vi "Dashboard Main.vi"() -> ()   [LabVIEW 2012]
uses:
  <vilib>/Rock Robotics/WPI/Camera/WPI_CameraImageSize.ctl
panel:
  out "Camera Image 3":T1(plugin-control)
  out "Camera Image":T1(plugin-control)
  # "Gatherer Camera"
  # "Shooter Camera"
  # "Team 195 - The CyberKnights"
  # "Screaming Knight Dashboard - 2012"
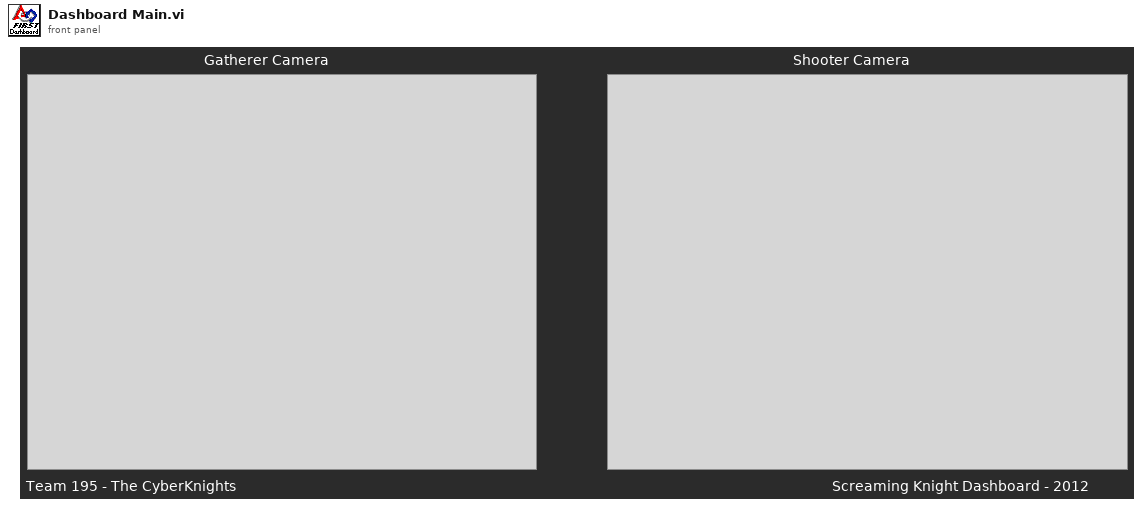
[diagram p1: front panel]
types:
  T1 = typedef "IMAQ Image.ctl" = refnum<image>
  T2 = typedef "Image Type" = u32
  T3 = typedef "WPI_CameraImageSize.ctl" = enum16{"640x480", "320x240", "160x120"}
  T4 = cluster{"fps":i32, "compression":i32, "Image Size":T3}
  T5 = cluster{"Desired Font (Application)":enum16{"User-specified Font", "Application Font", "System Font", "Dialog Font"}, "[User-specified Font]":cluster{"Font Name":string, "Size":i16, "Strikeout?":bool, "Italic?":bool, "Underline?":bool, "Outline?":bool, "Shadow?":bool, "Bold?":bool, "Rotation Angle":dbl}, "Horizontal Alignment":i16, "Vertical Alignment":i16}
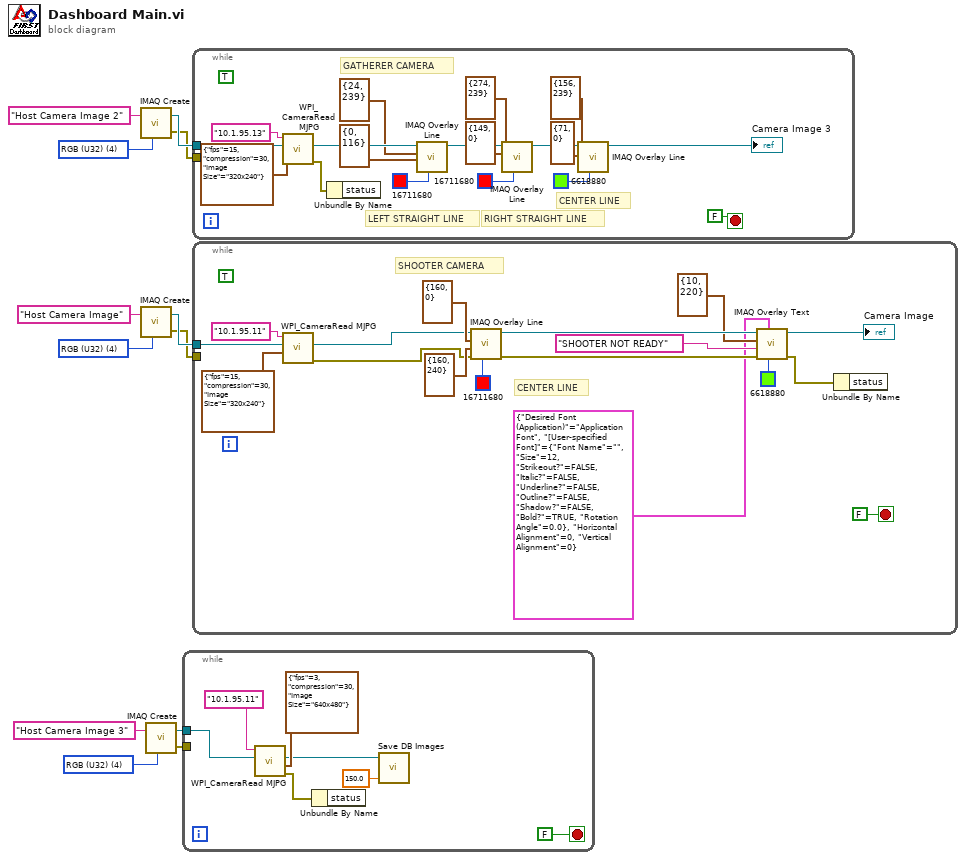
[diagram p0: block diagram]
diagram:
  w4 = T2 4 items=["Grayscale (U8)", "Grayscale (I16)", "Grayscale (SGL)", "Complex (CSG)", "RGB (U32)", "HSL (U32)", "RGB (U64)"] ("Image Type")
  w8 = T2 4 items=["Grayscale (U8)", "Grayscale (I16)", "Grayscale (SGL)", "Complex (CSG)", "RGB (U32)", "HSL (U32)", "RGB (U64)"] ("Image Type")
  w12 = T2 4 items=["Grayscale (U8)", "Grayscale (I16)", "Grayscale (SGL)", "Complex (CSG)", "RGB (U32)", "HSL (U32)", "RGB (U64)"] ("Image Type")
  n1 = call "IMAQ Create"("Image Name"="Host Camera Image 2", "Image Type"=w8) -> ("New Image"=w6:T1, "error out"=w5:errorcluster)  [unwired: 2 in, 1 out]
  n2 = call "IMAQ Create"("Image Name"="Host Camera Image", "Image Type"=w12) -> ("New Image"=w10:T1, "error out"=w9:errorcluster)  [unwired: 2 in, 1 out]
  n3 = call "IMAQ Create"("Image Name"="Host Camera Image 3", "Image Type"=w4) -> ("New Image"=w2:T1, "error out"=w1:errorcluster)  [unwired: 2 in, 1 out]
  n4 = while {
    tunnel: w2 -> [w18]
    tunnel: w1 -> [_]
    stop <- FALSE stop-if-true
    n5 = call <vilib>:"WPI_CameraRead MJPG.vi"("Camera Settings"=T4 {"fps"=3, "compression"=30, "Image Size"=enum."640x480"}, "Image"=w18, "address"="10.1.95.11") -> ("error out"=w19:errorcluster, "Image Out"=w15:T1)  [unwired: 6 in, 1 out]
    n6 = Unbundle By Name(w19) -> ()  [unwired: 1 out]
    n7 = call "Save DB Images.vi"("Images to Keep"=150.0, "Image"=w15) -> ()  [unwired: 2 in]
  }
  n8 = while {
    tunnel: w6 -> [w36]
    tunnel: w5 -> [_]
    stop <- FALSE stop-if-true
    (unwired) TRUE
    # "CENTER LINE"
    # "RIGHT STRAIGHT LINE"
    # "LEFT STRAIGHT LINE"
    # "GATHERER CAMERA"
    n9 = call <vilib>:"WPI_CameraRead MJPG.vi"("Camera Settings"=T4 {"fps"=15, "compression"=30, "Image Size"=enum."320x240"}, "Image"=w36, "address"="10.1.95.13") -> ("error out"=w34:errorcluster, "Image Out"=w33:T1)  [unwired: 6 in, 1 out]
    n10 = Unbundle By Name(w34) -> ()  [unwired: 1 out]
    n11 = call "IMAQ Overlay Line"("Color"=u32 16711680, "End Point"=cluster{"X":i32, "Y":i32} {"X"=0, "Y"=116}, "Start Point"=cluster{"X":i32, "Y":i32} {"X"=24, "Y"=239}, "Image"=w33) -> ("Image Out"=w32:T1)  [unwired: 6 in, 1 out]
    n12 = call "IMAQ Overlay Line"("Color"=u32 16711680, "End Point"=cluster{"X":i32, "Y":i32} {"X"=149, "Y"=0}, "Start Point"=cluster{"X":i32, "Y":i32} {"X"=274, "Y"=239}, "Image"=w32) -> ("Image Out"=w31:T1)  [unwired: 6 in, 1 out]
    n13 = call "IMAQ Overlay Line"("Color"=u32 6618880, "End Point"=cluster{"X":i32, "Y":i32} {"X"=71, "Y"=0}, "Start Point"=cluster{"X":i32, "Y":i32} {"X"=156, "Y"=239}, "Image"=w31) -> ("Image Out"=→"Camera Image 3":T1)  [unwired: 6 in, 1 out]
  }
  n14 = while {
    tunnel: w10 -> [w53]
    tunnel: w9 -> [_]
    stop <- FALSE stop-if-true
    (unwired) TRUE
    # "CENTER LINE"
    # "SHOOTER CAMERA"
    n15 = call <vilib>:"WPI_CameraRead MJPG.vi"("Camera Settings"=T4 {"fps"=15, "compression"=30, "Image Size"=enum."320x240"}, "Image"=w53, "address"="10.1.95.11") -> ("error out"=w46:errorcluster, "Image Out"=w47:T1)  [unwired: 6 in, 1 out]
    n16 = call "IMAQ Overlay Line"("Color"=u32 16711680, "error in (no error)"=w46, "End Point"=cluster{"X":i32, "Y":i32} {"X"=160, "Y"=240}, "Start Point"=cluster{"X":i32, "Y":i32} {"X"=160, "Y"=0}, "Image"=w47) -> ("error out"=w42:errorcluster, "Image Out"=w45:T1)  [unwired: 5 in]
    n17 = call "IMAQ Overlay Text"("Text Color (black)"=u32 6618880, "Font, Size & Style"=T5 {"Desired Font (Application)"=enum."Application Font", "[User-specified Font]"={"Font Name"="", "Size"=12, "Strikeout?"=FALSE, "Italic?"=FALSE, "Underline?"=FALSE, "Outline?"=FALSE, "Shadow?"=FALSE, "Bold?"=TRUE, "Rotation Angle"=0.0}, "Horizontal Alignment"=0, "Vertical Alignment"=0}, "error in (no error)"=w42, "String"="SHOOTER NOT READY", "Origin"=cluster{"X":i32, "Y":i32} {"X"=10, "Y"=220}, "Image"=w45) -> ("error out"=w41:errorcluster, "Image Out"=→"Camera Image":T1)  [unwired: 4 in]
    n18 = Unbundle By Name(w41) -> ()  [unwired: 1 out]
  }
